vi "Home motors.vi"(8 "error in":errorcluster, 9 "Home direction (M2)":T1=1 items=["", "Forward", "Backward"], 10 "Home direction (M1)":T1=1 items=["", "Forward", "Backward"], 11 "Module ID":i32=-1) -> (0 "error out":errorcluster)   [LabVIEW 2020, in "Arduino-Adafruit stepper.lvlib"]
doc: "Request to move motors to home position. Home position can be especified for each motor.\n_____\nCreated using DQMH Event Scripter 7.0.1.1316."
uses:
  Arduino-Adafruit stepper.lvlib
  Arduino stepper library/Public/Controls/Motor direction.ctl
  Home motors Argument--cluster.ctl
  Arduino stepper library/Control de MaP.lvlib
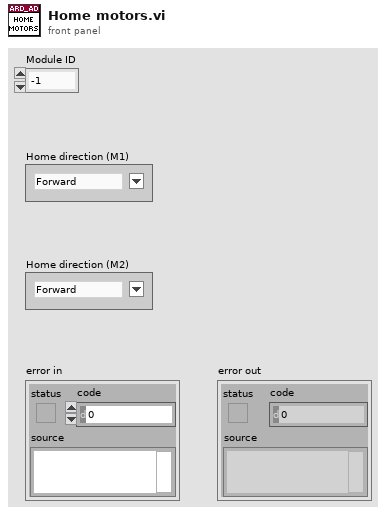
[diagram p1: front panel]
types:
  T1 = typedef "Control de MaP.lvlib/Motor direction.ctl" = u8
  T2 = typedef "Arduino-Adafruit stepper.lvlib/Home motors Argument--cluster.ctl" = cluster{"Module ID":i32, "Home direction (M1)":T1, "Home direction (M2)":T1}
  T3 = typedef "Arduino-Adafruit stepper.lvlib/Request Events--cluster.ctl" = cluster{"Stop Module":refnum<user-event>, "Show Panel":refnum<user-event>, "Hide Panel":refnum<user-event>, "Show Diagram":refnum<user-event>, "Get Module Execution Status":refnum<user-event>, "Initialize Arduino":refnum<user-event>, "Connect":refnum<user-event>, "Disconnect":refnum<user-event>, "Init motors":refnum<user-event>, "Home motors":refnum<user-event>}
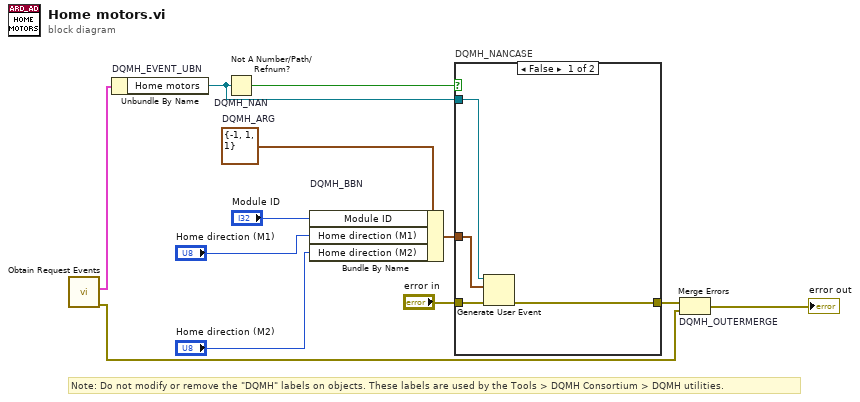
[diagram p0: block diagram]
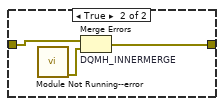
[diagram p2: hidden frame]
diagram:
  w6 = T2 {"Module ID"=-1, "Home direction (M1)"=1, "Home direction (M2)"=1}  # DQMH_ARG
  # "Note: Do not modify or remove the \"DQMH\" labels on objects. These labels are used by the Tools > DQMH Consortium > DQMH utilities."
  n1 = call "Obtain Request Events.vi"() -> ("error out"=w2:errorcluster, "Arduino-Adafruit stepper Request Events"=w1:T3)  [unwired: 10 in]
  n2 = Unbundle By Name "DQMH_EVENT_UBN"(w1) -> ("Home motors"=w8:refnum<user-event>)
  n3 = Not A Number/Path/Refnum? "DQMH_NAN"(number/path/refnum=w8) -> (NaN/Path/Refnum?=w9:bool)
  n4 = Bundle By Name "DQMH_BBN"(cluster=w6, "Module ID"="Module ID", "Home direction (M1)"="Home direction (M1)", "Home direction (M2)"="Home direction (M2)") -> (w10:T2)
  n5 = case "DQMH_NANCASE" shown="False" w9 {
    tunnel: "error in" -> [w16 w19]
    tunnel: [w15 w18] -> w7
    tunnel: w8 -> [w14 _]
    tunnel: w10 -> [w13 _]
    frame False {
      n6 = Generate User Event(user event=w14, event data cluster=w13, error in=w16) -> (error out=w15:errorcluster)  [unwired: 1 in, 1 out]
    }
    frame True {
      n7 = call "Module Not Running--error.vi"() -> ("error out"=w17:errorcluster)  [unwired: 11 in]
      n8 = Merge Errors "DQMH_INNERMERGE"(w19, w17) -> (w18:errorcluster)
    }
  }
  n9 = Merge Errors "DQMH_OUTERMERGE"(w7, w2) -> (→"error out":errorcluster)
